vi "Start and Wait for Event.vi"(7 "error in":errorcluster, 10 "Start and wait event config":T1={"Source Ganged Session Out"={"Ganged Config"=enum."Series", "Session List"=[], "Session Mode"=[], "Channel"=[]}, "Load Ganged Session Out"={"Ganged Config"=enum."Series", "Session List"=[], "Session Mode"=[], "Channel"=[]}, "Source session out"="", "Load session out"="", "event"=1030, "Source channel name"="", "Load channel name"="", "Load Source ON/OFF"=enum."SOURCE AND LOAD OFF", "Load ganged/single"=FALSE, "Source ganged/single"=FALSE} {"event" items=["Source Complete Event"=1030, "Measure Complete Event"=1031, "Sequence Iteration Complete Event"=1032, "Sequence Engine Done Event"=1033, "Pulse Complete Event"=1051, "Ready For Pulse Trigger Event"=1052]}) -> (0 "error out":errorcluster, 3 "Start and wait event result":T1={"Source Ganged Session Out"={"Ganged Config"=enum."Series", "Session List"=[], "Session Mode"=[], "Channel"=[]}, "Load Ganged Session Out"={"Ganged Config"=enum."Series", "Session List"=[], "Session Mode"=[], "Channel"=[]}, "Source session out"="", "Load session out"="", "event"=1030, "Source channel name"="", "Load channel name"="", "Load Source ON/OFF"=enum."SOURCE AND LOAD OFF", "Load ganged/single"=FALSE, "Source ganged/single"=FALSE} {"event" items=["Source Complete Event"=1030, "Measure Complete Event"=1031, "Sequence Iteration Complete Event"=1032, "Sequence Engine Done Event"=1033, "Pulse Complete Event"=1051, "Ready For Pulse Trigger Event"=1052]})   [LabVIEW 2021]
uses:
  controls/Start and Wait for Event.ctl
  channel ganging/shared subVIs/ctl/NIDCPower_channel_ganging - ctl - ganged session.ctl
  channel ganging/shared subVIs/ctl/NIDCPower_channel_ganging - ctl - ganged config.ctl
  channel ganging/shared subVIs/ctl/NIDCPower_channel_ganging - ctl - channel mode.ctl
  <instrlib>/niDCPower/nidcpower.llb/niDCPower Wait For Event - Event.ctl
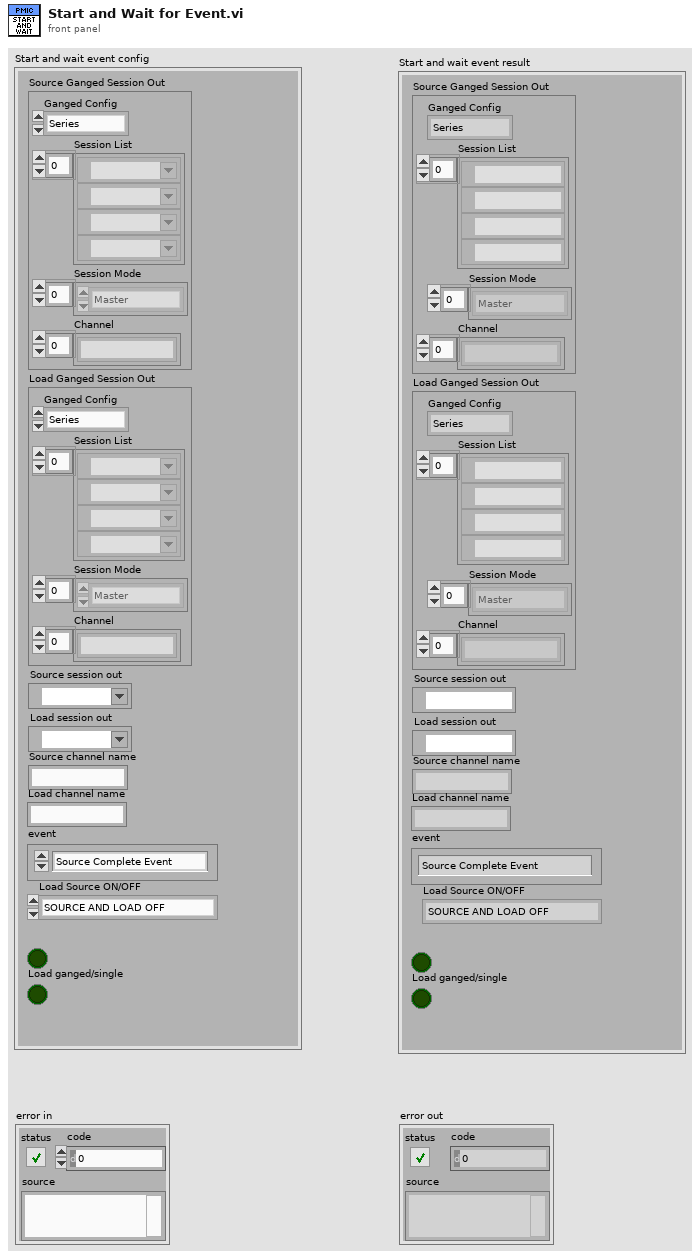
[diagram p1: front panel]
types:
  T1 = typedef "Start and Wait for Event.ctl" = cluster{"Source Ganged Session Out":T2, "Load Ganged Session Out":T2, "Source session out":refnum<k15>, "Load session out":refnum<k15>, "event":T5, "Source channel name":string, "Load channel name":string, "Load Source ON/OFF":enum16{"SOURCE AND LOAD OFF", "SOURCE ON", "LOAD ON", "SOURCE AND LAOD ON"}, "Load ganged/single":bool, "Source ganged/single":bool}
  T2 = typedef "NIDCPower_channel_ganging - ctl - ganged session.ctl" = cluster{"Ganged Config":T3, "Session List":refnum<k15>[], "Session Mode":T4[], "Channel":string[]}
  T3 = typedef "NIDCPower_channel_ganging - ctl - ganged config.ctl" = enum32{"Series", "Parallel", "Manual"}
  T4 = typedef "NIDCPower_channel_ganging - ctl - channel mode.ctl" = enum32{"Master", "Slave", "Slave - Inverted"}
  T5 = typedef "niDCPower Wait For Event - Event.ctl" = i32
  T6 = enum16{"SOURCE AND LOAD OFF", "SOURCE ON", "LOAD ON", "SOURCE AND LAOD ON"}
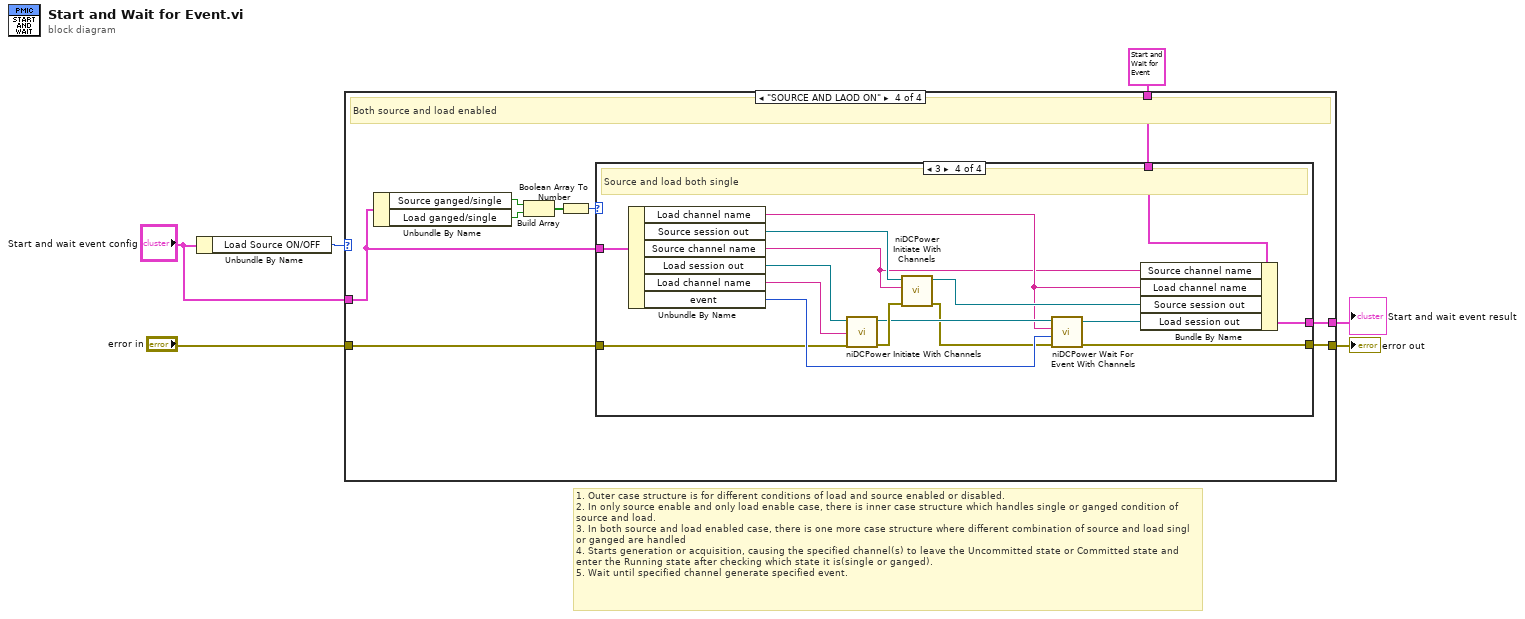
[diagram p0: block diagram]
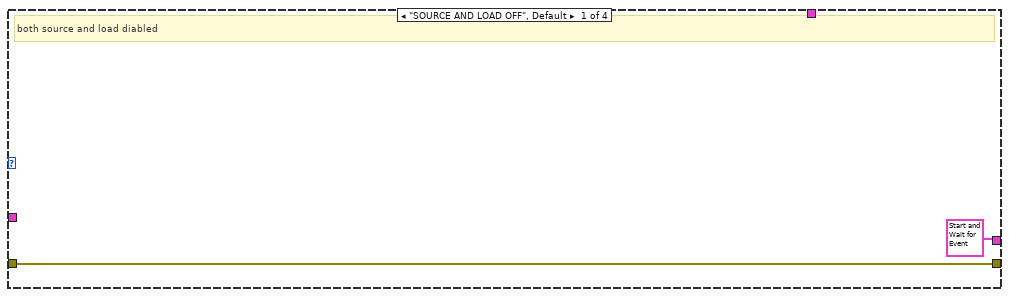
[diagram p2: hidden frame]
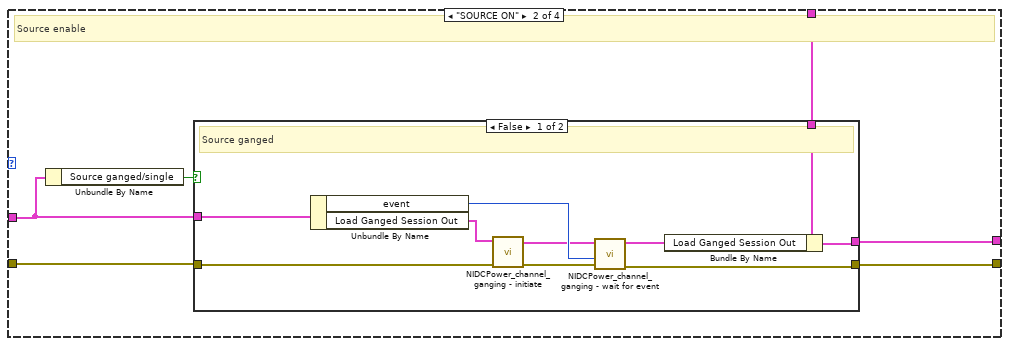
[diagram p3: hidden frame]
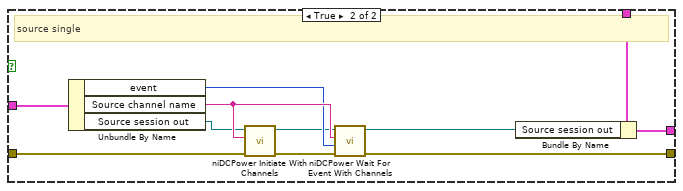
[diagram p4: hidden frame]
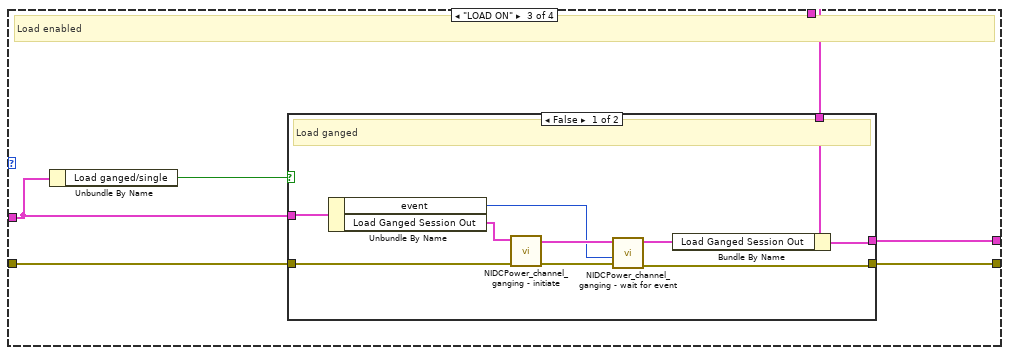
[diagram p5: hidden frame]
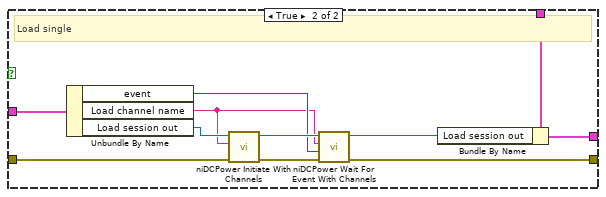
[diagram p6: hidden frame]
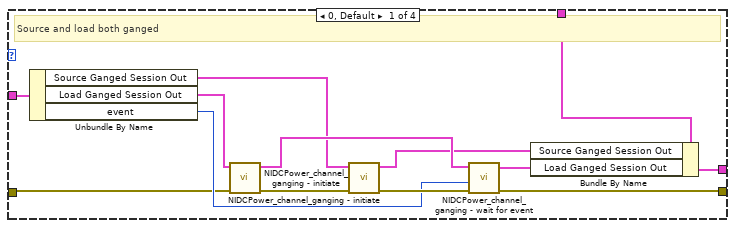
[diagram p7: hidden frame]
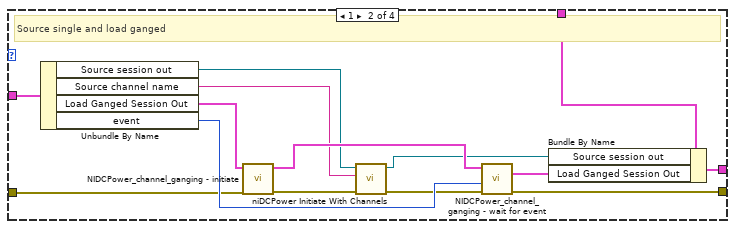
[diagram p8: hidden frame]
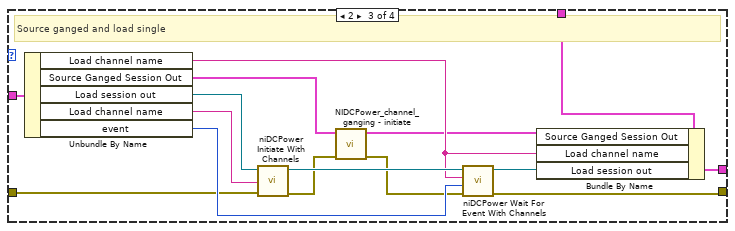
[diagram p9: hidden frame]
diagram:
  # "1. Outer case structure is for different conditions of load and source enabled or disabled.\n2. In only source enable and only load enable case, there is inner case structure which handles single or ganged condition of source and load. \n3. In both source and load enabled case, there is one more case structure where different combination of source and load singl or ganged are handled\n4. Starts generation or acquisition, causing the specified channel(s) to leave the Uncommitted state or Committed state and enter the Running state after checking which state it is(single or ganged).\n5. Wait until specified channel generate specified event."
  n1 = Unbundle By Name("Start and wait event config") -> ("Load Source ON/OFF"=w6:T6)
  n2 = case shown="\"SOURCE AND LAOD ON\"" w6 {
    tunnel: "Start and wait event config" -> [_ w13 w38 w67]
    tunnel: "error in" -> [w8 w12 w40 w66]
    tunnel: [w8 w11 w39 w65] -> w4
    tunnel: T1 {"Source Ganged Session Out"={"Ganged Config"=enum."Series", "Session List"=[], "Session Mode"=[], "Channel"=[]}, "Load Ganged Session Out"={"Ganged Config"=enum."Series", "Session List"=[], "Session Mode"=[], "Channel"=[]}, "Source session out"="", "Load session out"="", "event"=1030, "Source channel name"="", "Load channel name"="", "Load Source ON/OFF"=enum."SOURCE AND LOAD OFF", "Load ganged/single"=FALSE, "Source ganged/single"=FALSE} ("Start and wait event config 2") -> [_ w10 w37 w64]
    tunnel: [T1 {"Source Ganged Session Out"={"Ganged Config"=enum."Series", "Session List"=[], "Session Mode"=[], "Channel"=[]}, "Load Ganged Session Out"={"Ganged Config"=enum."Series", "Session List"=[], "Session Mode"=[], "Channel"=[]}, "Source session out"="", "Load session out"="", "event"=1030, "Source channel name"="", "Load channel name"="", "Load Source ON/OFF"=enum."SOURCE AND LOAD OFF", "Load ganged/single"=FALSE, "Source ganged/single"=FALSE} ("Start and wait event config 2") w9 w36 w63] -> w1
    frame "SOURCE AND LOAD OFF", Default {
      # "both source and load diabled"
    }
    frame "SOURCE ON" {
      # "Source enable"
      n3 = Unbundle By Name(w13) -> ("Source ganged/single"=w14:bool)
      n4 = case shown="False" w14 {
        tunnel: w13 -> [w15 w29]
        tunnel: w12 -> [w19 w28]
        tunnel: [w18 w27] -> w11
        tunnel: w10 -> [w16 w26]
        tunnel: [w17 w25] -> w9
        frame False {
          # "Source ganged"
          n5 = Unbundle By Name(w15) -> ("event"=w23:T5, "Load Ganged Session Out"=w22:T2)
          n6 = call "NIDCPower_channel_ganging - initiate.vi"("error in (no error)"=w19, "Ganged Session In"=w22) -> ("error out"=w20:errorcluster, "Ganged Session Out"=w21:T2)  [unwired: 8 in]
          n7 = call "NIDCPower_channel_ganging - wait for event.vi"("error in (no error)"=w20, "event"=w23, "Ganged Session in"=w21) -> ("error out"=w18:errorcluster, "Ganged Session Out"=w24:T2)  [unwired: 7 in]
          n8 = Bundle By Name(cluster=w16, "Load Ganged Session Out"=w24) -> (w17:T1)
        }
        frame True {
          # "source single"
          n9 = Unbundle By Name(w29) -> ("event"=w32:T5, "Source channel name"=w34:string, "Source session out"=w33:refnum<k15>)
          n10 = call <instrlib>:"niDCPower Initiate With Channels.vi"("error in (no error)"=w28, "channel name"=w34, "instrument handle"=w33) -> ("error out"=w30:errorcluster, "instrument handle out"=w31:refnum<k15>)  [unwired: 7 in]
          n11 = call <instrlib>:"niDCPower Wait For Event With Channels.vi"("error in (no error)"=w30, "event"=w32, "channel name"=w34, "instrument handle"=w31) -> ("error out"=w27:errorcluster, "instrument handle out"=w35:refnum<k15>)  [unwired: 6 in]
          n12 = Bundle By Name(cluster=w26, "Source session out"=w35) -> (w25:T1)
        }
      }
    }
    frame "LOAD ON" {
      # "Load enabled"
      n13 = Unbundle By Name(w38) -> ("Load ganged/single"=w41:bool)
      n14 = case shown="False" w41 {
        tunnel: w38 -> [w49 w60]
        tunnel: w40 -> [w46 w59]
        tunnel: [w45 w58] -> w39
        tunnel: w37 -> [w44 w54]
        tunnel: [w42 w52] -> w36
        frame False {
          # "Load ganged"
          n15 = Unbundle By Name(w49) -> ("event"=w47:T5, "Load Ganged Session Out"=w48:T2)
          n16 = call "NIDCPower_channel_ganging - initiate.vi"("error in (no error)"=w46, "Ganged Session In"=w48) -> ("error out"=w51:errorcluster, "Ganged Session Out"=w50:T2)  [unwired: 8 in]
          n17 = call "NIDCPower_channel_ganging - wait for event.vi"("error in (no error)"=w51, "event"=w47, "Ganged Session in"=w50) -> ("error out"=w45:errorcluster, "Ganged Session Out"=w43:T2)  [unwired: 7 in]
          n18 = Bundle By Name(cluster=w44, "Load Ganged Session Out"=w43) -> (w42:T1)
        }
        frame True {
          # "Load single"
          n19 = Unbundle By Name(w60) -> ("event"=w57:T5, "Load channel name"=w55:string, "Load session out"=w56:refnum<k15>)
          n20 = call <instrlib>:"niDCPower Initiate With Channels.vi"("error in (no error)"=w59, "channel name"=w55, "instrument handle"=w56) -> ("error out"=w62:errorcluster, "instrument handle out"=w61:refnum<k15>)  [unwired: 7 in]
          n21 = call <instrlib>:"niDCPower Wait For Event With Channels.vi"("error in (no error)"=w62, "event"=w57, "channel name"=w55, "instrument handle"=w61) -> ("error out"=w58:errorcluster, "instrument handle out"=w53:refnum<k15>)  [unwired: 6 in]
          n22 = Bundle By Name(cluster=w54, "Load session out"=w53) -> (w52:T1)
        }
      }
    }
    frame "SOURCE AND LAOD ON" {
      # "Both source and load enabled"
      n23 = Unbundle By Name(w67) -> ("Source ganged/single"=w71:bool, "Load ganged/single"=w70:bool)
      n24 = Build Array(w71, w70) -> (w69:bool[])
      n25 = Boolean Array To Number(Boolean array=w69) -> (number=w68:u32)
      n26 = case shown="3" w68 {
        tunnel: w67 -> [w76 w87 w99 w118]
        tunnel: w66 -> [w75 w93 w107 w117]
        tunnel: [w74 w94 w106 w116] -> w65
        tunnel: w64 -> [w72 w86 w104 w115]
        tunnel: [w73 w85 w105 w114] -> w63
        frame 0, Default {
          # "Source and load both ganged"
          n27 = Unbundle By Name(w76) -> ("Source Ganged Session Out"=w81:T2, "Load Ganged Session Out"=w80:T2, "event"=w79:T5)
          n28 = call "NIDCPower_channel_ganging - initiate.vi"("error in (no error)"=w75, "Ganged Session In"=w80) -> ("error out"=w82:errorcluster, "Ganged Session Out"=w84:T2)  [unwired: 8 in]
          n29 = call "NIDCPower_channel_ganging - initiate.vi"("error in (no error)"=w82, "Ganged Session In"=w81) -> ("error out"=w83:errorcluster, "Ganged Session Out"=w78:T2)  [unwired: 8 in]
          n30 = call "NIDCPower_channel_ganging - wait for event.vi"("error in (no error)"=w83, "event"=w79, "Ganged Session in"=w84) -> ("error out"=w74:errorcluster, "Ganged Session Out"=w77:T2)  [unwired: 7 in]
          n31 = Bundle By Name(cluster=w72, "Source Ganged Session Out"=w78, "Load Ganged Session Out"=w77) -> (w73:T1)
        }
        frame 1 {
          # "Source single and load ganged"
          n32 = Unbundle By Name(w87) -> ("Source session out"=w89:refnum<k15>, "Source channel name"=w88:string, "Load Ganged Session Out"=w97:T2, "event"=w96:T5)
          n33 = call "NIDCPower_channel_ganging - initiate.vi"("error in (no error)"=w93, "Ganged Session In"=w97) -> ("error out"=w92:errorcluster, "Ganged Session Out"=w98:T2)  [unwired: 8 in]
          n34 = call <instrlib>:"niDCPower Initiate With Channels.vi"("error in (no error)"=w92, "channel name"=w88, "instrument handle"=w89) -> ("error out"=w91:errorcluster, "instrument handle out"=w90:refnum<k15>)  [unwired: 7 in]
          n35 = call "NIDCPower_channel_ganging - wait for event.vi"("error in (no error)"=w91, "event"=w96, "Ganged Session in"=w98) -> ("error out"=w94:errorcluster, "Ganged Session Out"=w95:T2)  [unwired: 7 in]
          n36 = Bundle By Name(cluster=w86, "Source session out"=w90, "Load Ganged Session Out"=w95) -> (w85:T1)
        }
        frame 2 {
          # "Source ganged and load single"
          n37 = Unbundle By Name(w99) -> ("Load channel name"=w108:string, "Source Ganged Session Out"=w103:T2, "Load session out"=w112:refnum<k15>, "Load channel name"=w111:string, "event"=w113:T5)
          n38 = call <instrlib>:"niDCPower Initiate With Channels.vi"("error in (no error)"=w107, "channel name"=w111, "instrument handle"=w112) -> ("error out"=w101:errorcluster, "instrument handle out"=w110:refnum<k15>)  [unwired: 7 in]
          n39 = call "NIDCPower_channel_ganging - initiate.vi"("error in (no error)"=w101, "Ganged Session In"=w103) -> ("error out"=w100:errorcluster, "Ganged Session Out"=w102:T2)  [unwired: 8 in]
          n40 = call <instrlib>:"niDCPower Wait For Event With Channels.vi"("error in (no error)"=w100, "event"=w113, "channel name"=w108, "instrument handle"=w110) -> ("error out"=w106:errorcluster, "instrument handle out"=w109:refnum<k15>)  [unwired: 6 in]
          n41 = Bundle By Name(cluster=w104, "Source Ganged Session Out"=w102, "Load channel name"=w108, "Load session out"=w109) -> (w105:T1)
        }
        frame 3 {
          # "Source and load both single"
          n42 = Unbundle By Name(w118) -> ("Load channel name"=w120:string, "Source session out"=w127:refnum<k15>, "Source channel name"=w119:string, "Load session out"=w126:refnum<k15>, "Load channel name"=w125:string, "event"=w128:T5)
          n43 = call <instrlib>:"niDCPower Initiate With Channels.vi"("error in (no error)"=w117, "channel name"=w125, "instrument handle"=w126) -> ("error out"=w129:errorcluster, "instrument handle out"=w124:refnum<k15>)  [unwired: 7 in]
          n44 = call <instrlib>:"niDCPower Initiate With Channels.vi"("error in (no error)"=w129, "channel name"=w119, "instrument handle"=w127) -> ("error out"=w123:errorcluster, "instrument handle out"=w121:refnum<k15>)  [unwired: 7 in]
          n45 = call <instrlib>:"niDCPower Wait For Event With Channels.vi"("error in (no error)"=w123, "event"=w128, "channel name"=w120, "instrument handle"=w124) -> ("error out"=w116:errorcluster, "instrument handle out"=w122:refnum<k15>)  [unwired: 6 in]
          n46 = Bundle By Name(cluster=w115, "Source channel name"=w119, "Load channel name"=w120, "Source session out"=w121, "Load session out"=w122) -> (w114:T1)
        }
      }
    }
  }
  "error out" <- w4
  "Start and wait event result" <- w1
